vi "Get Target Train Field.vi"(8 "Train to Field":dbl[unit]=7.0, 9 "Original Field":dbl[unit], 10 "going up?":bool=TRUE, 11 "Power Supply in":refnum<class "Power Supply.lvclass">) -> (2 "Target Field":dbl[unit], 3 "Power Supply Out":refnum<class "Power Supply.lvclass">)   [LabVIEW 2017, in "Power Supply.lvclass"]
uses:
  Power Supply.lvclass
  Power Supply.lvclass/Power Supply.ctl
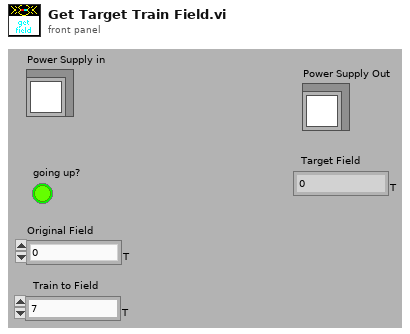
[diagram p1: front panel]
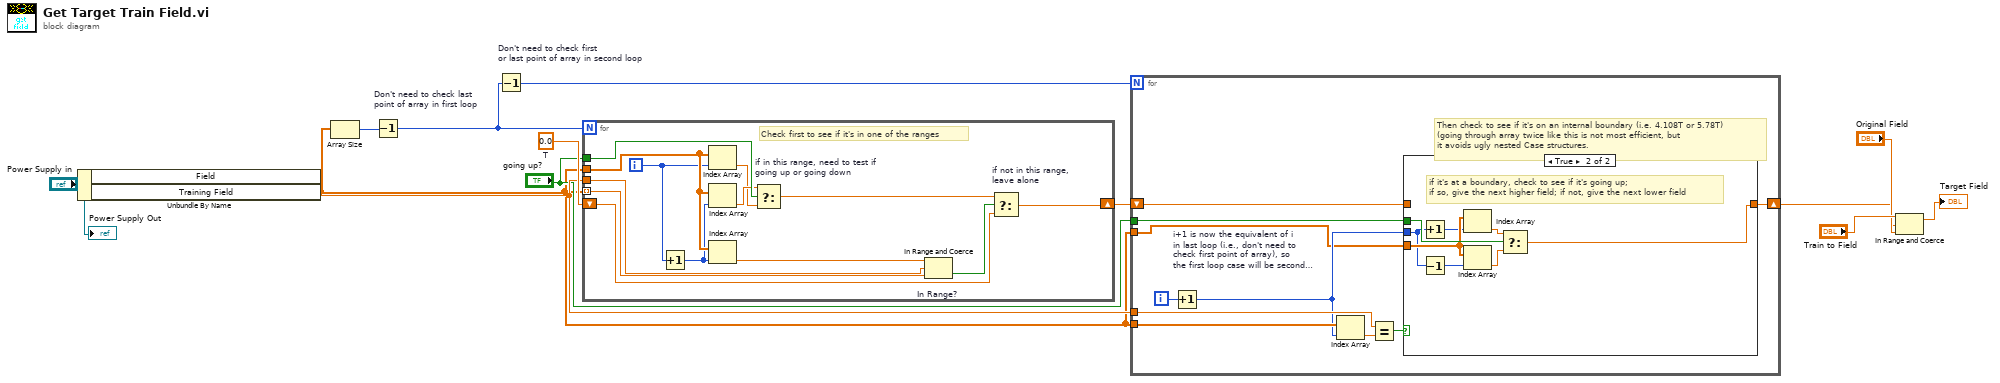
[diagram p0: block diagram]
diagram:
  w11 = dbl[unit] 0.0  # T
  n1 = Unbundle By Name("Power Supply in") -> ("Field"=w8:dbl[unit], "Training Field"=w5:dbl[unit][])
  n2 = Array Size(array=w5) -> (size(s)=w12:i32)
  n3 = Decrement "Don't need to check last \npoint of array in first loop"(x=w12) -> (x-1=w9:i32)
  n4 = Decrement "Don't need to check first\nor last point of array in second loop"(x=w9) -> (x-1=w7:i32)
  n5 = for {
    N: w9 -> [_]
    tunnel: w8 -> [w25]
    tunnel: w5 -> [w19]
    tunnel: w5 -> [w24] mode=indexing
    shift-right: [w22] -> w10
    shift-left: w11 -> [w21]
    tunnel: "going up?" -> [w20]
    i -> [w17]
    # "Check first to see if it's in one of the ranges"
    n6 = Increment(x=w17) -> (x+1=w18:i32)
    n7 = Index Array(array=w19, index=w17) -> (element=w15:dbl[unit])
    n8 = Index Array(array=w19, index=w18) -> (element=w16:dbl[unit])
    n9 = Index Array(array=w19, index=w18) -> (element=w26:dbl[unit])
    n10 = Select "if in this range, need to test if \ngoing up or going down"(t=w16, s=w20, f=w15) -> (s? t:f=w14:dbl[unit])
    n11 = In Range and Coerce "In Range?"(upper limit=w26, x=w25, lower limit=w24) -> (In Range?=w23:bool)  [unwired: 1 out]
    n12 = Select "if not in this range,\nleave alone"(t=w14, s=w23, f=w21) -> (s? t:f=w22:dbl[unit])
  }
  n13 = for {
    N: w7 -> [_]
    tunnel: w8 -> [w33]
    tunnel: w5 -> [w31]
    shift-right: [w35] -> w1
    shift-left: w10 -> [w34]
    tunnel: "going up?" -> [w28]
    tunnel: w5 -> [w27]
    i -> [w36]
    # "Then check to see if it's on an internal boundary (i.e. 4.108T or 5.78T)\n(going through array twice like this is not most efficient, but\nit avoids ugly nested Case structures."
    n14 = Increment "i+1 is now the equivalent of i\nin last loop (i.e., don't need to \ncheck first point of array), so \nthe first loop case will be second\npoint"(x=w36) -> (x+1=w29:i32)
    n15 = Index Array(array=w31, index=w29) -> (element=w30:dbl[unit])
    n16 = Equal?(x=w33, y=w30) -> (x = y?=w32:bool)
    n17 = case shown="True" w32 {
      tunnel: [w37 w40] -> w35
      tunnel: w34 -> [w37 _]
      tunnel: w29 -> [_ w39]
      tunnel: w28 -> [_ w42]
      tunnel: w27 -> [_ w41]
      frame False {
        # "if not at a boundary, just use the value determined \nfrom the range business of the last loop"
      }
      frame True {
        # "if it's at a boundary, check to see if it's going up; \nif so, give the next higher field; if not, give the next lower field"
        n18 = Increment(x=w39) -> (x+1=w38:i32)
        n19 = Decrement(x=w39) -> (x-1=w45:i32)
        n20 = Index Array(array=w41, index=w38) -> (element=w44:dbl[unit])
        n21 = Index Array(array=w41, index=w45) -> (element=w43:dbl[unit])
        n22 = Select(t=w44, s=w42, f=w43) -> (s? t:f=w40:dbl[unit])
      }
    }
  }
  n23 = In Range and Coerce(upper limit="Train to Field", x=w1, lower limit="Original Field") -> (coerced(x)=→"Target Field":dbl[unit])  [unwired: 1 out]
  "Power Supply Out" <- "Power Supply in"
